vi "FTW-Actor-Log-Event.vi"(0 "FTW Actor Instance":refnum<class "FTW-Actor-Instance.lvclass">, 5 "Event Type":string, 7 "Event Data":string, 11 "error in":errorcluster) -> (4 "FTW Actor Instance out":refnum<class "FTW-Actor-Instance.lvclass">, 15 "error out":errorcluster)   [LabVIEW 2015, in "FTW-Actor-Instance.lvclass"]
uses:
  FTW-Actor-Instance.lvclass
  FTW-Actor-Instance.lvclass/FTW-Actor-Instance.ctl
panel:
  # "Inputs"
  # "Outputs"
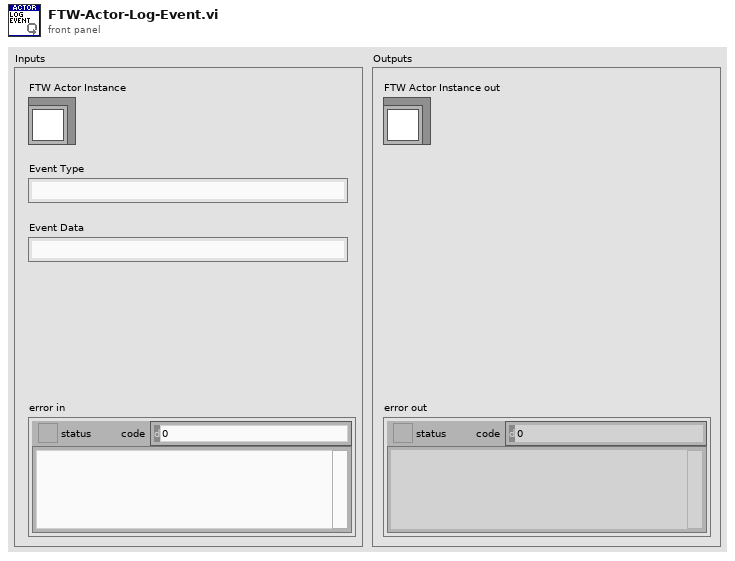
[diagram p1: front panel]
types:
  T1 = typedef "FTW-Type-Actor-Connector.ctl" = refnum<data-value>
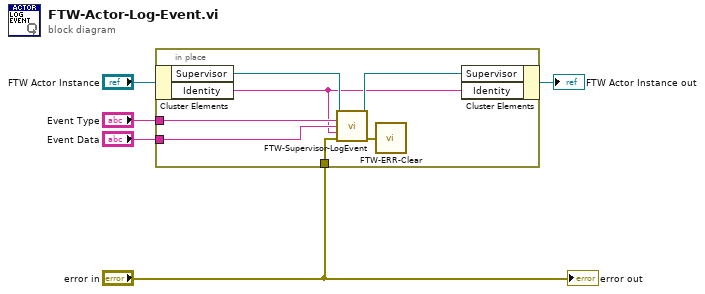
[diagram p0: block diagram]
diagram:
  n1 = in-place {
    in-place-border: "error in" -> [w12]
    in-place-border: "Event Type" -> [w9]
    in-place-border: "Event Data" -> [w8]
    n2 = in-place-cluster #1("FTW Actor Instance") -> ("Supervisor"=w11:T1, "Identity"=w7:string)
    n3 = call "FTW-Supervisor-LogEvent.vi"("FTW Supervisor Connection"=w11, "Event Type"=w9, "Event Data"=w8, "Source (unwired for call chain)"=w7, "error in"=w12) -> ("FTW Supervisor Connection out"=w10:T1, "error out"=w6:errorcluster)  [unwired: 9 in]
    n4 = call "FTW-ERR-Clear.vi"("error to snuff"=w6) -> ()  [unwired: 1 out]
    n5 = in-place-cluster #1("Supervisor"=w10, "Identity"=w7) -> (→"FTW Actor Instance out":refnum<class "FTW-Actor-Instance.lvclass">)
  }
  "error out" <- "error in"
